vi "FindItemByTag.vi"(8 "error in (no error)":errorcluster, 10 "Tag":string, 11 "MGI_ToolStrip in":refnum<class "MGI_ToolStrip.lvclass">) -> (0 "error out":errorcluster, 2 "ToolStripItem":refnum<k24>, 3 "MGI_ToolStrip out":refnum<class "MGI_ToolStrip.lvclass">)   [LabVIEW 2019, in "MGI_ToolStrip.lvclass"]
uses:
  MGI_ToolStrip.lvclass
  System.Windows.Forms
  MGI_ToolStrip.lvclass/MGI_ToolStrip.ctl
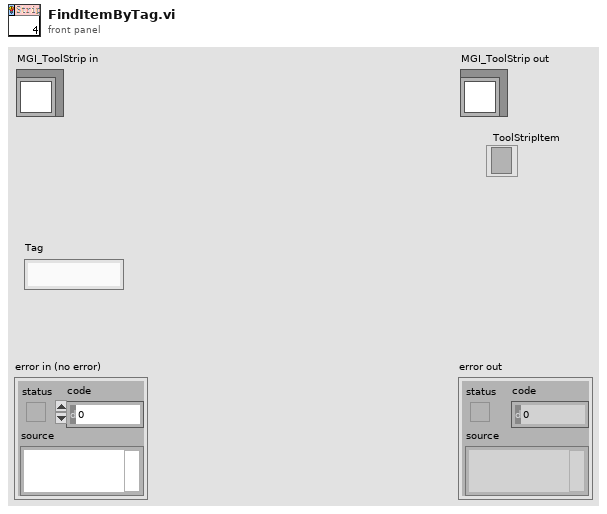
[diagram p1: front panel]
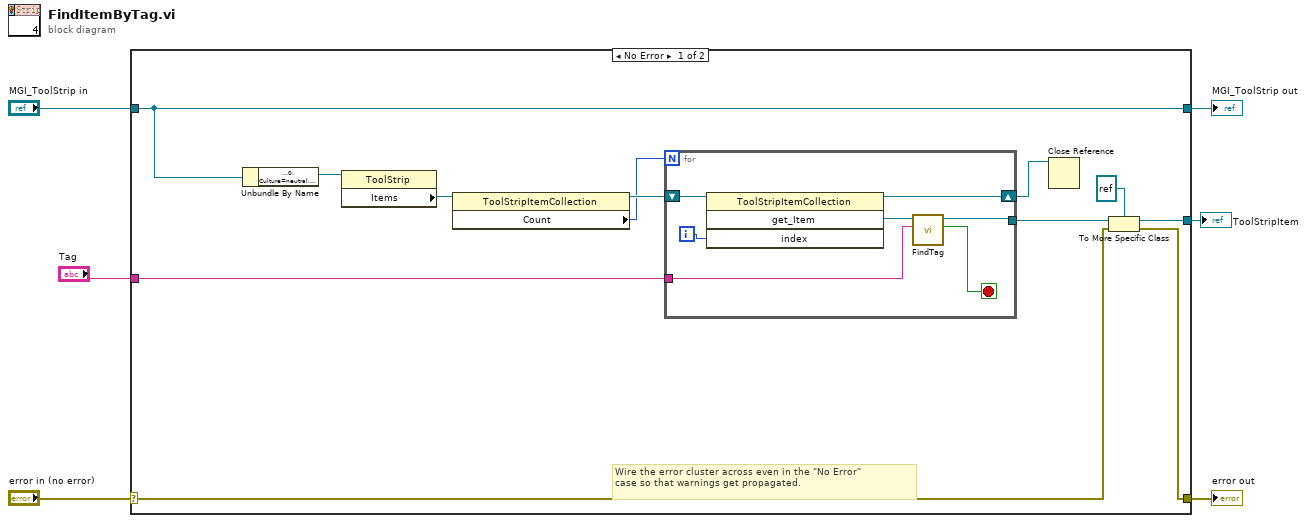
[diagram p0: block diagram]
diagram:
  n1 = case shown="No Error" "error in (no error)" {
    selector: "error in (no error)" -> [w10 w27]
    tunnel: [w9 w27] -> w5
    tunnel: [w18 w26] -> w3
    tunnel: "MGI_ToolStrip in" -> [w18 w26]
    tunnel: "Tag" -> [w13 _]
    tunnel: [w7 _] -> w1
    frame No Error {
      # "Wire the error cluster across even in the \"No Error\"\ncase so that warnings get propagated."
      n2 = Unbundle By Name(w18) -> ("ToolStrip"=w16:refnum<k24>)
      n3 = property class="ToolStrip"(reference=w16) -> ("Items"=w17:refnum<k24>)  [unwired: 1 in, 2 out]
      n4 = property class="ToolStripItemCollection"(reference=w17) -> (reference out=w15:refnum<k24>, "Count"=w14:i32)  [unwired: 1 in, 1 out]
      n5 = for {
        N: w14 -> [_]
        tunnel: w13 -> [w22]
        shift-right: [w20] -> w12
        shift-left: w15 -> [w25]
        tunnel: [w19] -> w11
        i -> [w24]
        stop <- w21 stop-if-true
        n6 = invoke class="ToolStripItemCollection" method="get_Item"(reference=w25, "index"=w24) -> (reference out=w20:refnum<k24>, "get_Item"=w23:refnum<k24>)  [unwired: 2 in, 2 out]
        n7 = call "FindTag.vi"("Tag"=w22, "ToolStripItem"=w23) -> ("Found"=w21:bool, "ToolStripItem out"=w19:refnum<k24>)  [unwired: 7 in, 1 out]
      }
      n8 = Close Reference(reference=w12) -> ()  [unwired: 1 in, 1 out]
      n9 = To More Specific Class(target class=refnum<k24> refnum ("new reference"), reference=w11, error in=w10) -> (specific class reference=w7:refnum<k24>, error out=w9:errorcluster)
    }
    frame Error {
    }
  }
  "error out" <- w5
  "MGI_ToolStrip out" <- w3
  "ToolStripItem" <- w1
